vi "TH_Bladmögelvarning.vi"(4 "Bladmögelvarning":T1={"Tid (Timmar)"=5.0, "Grader (°C)"=15.0, "Fuktighet (%)"=80.0} {"Fuktighet (%)" min=0.0 max=100.0 format="%.1f"; "Grader (°C)" min=-25.0 max=85.0 format="%.1f"; "Tid (Timmar)" min=0.01 format="%.2f"}, 6 "Humidities In":dbl[](array[numeric]) format="%.2f", 7 "Temperatures In":dbl[](array[numeric]) format="%.2f") -> (3 "Bladmägelvarning (T/F)":bool)   [LabVIEW 2014]
panel:
  in  "Startflag":bool
  out "Starttid (sec)":dbl
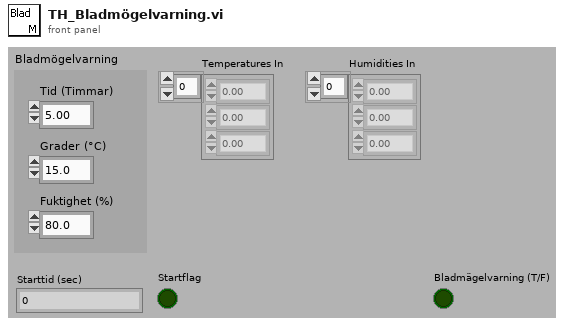
[diagram p1: front panel]
types:
  T1 = cluster{"Tid (Timmar)":dbl, "Grader (°C)":dbl, "Fuktighet (%)":dbl}
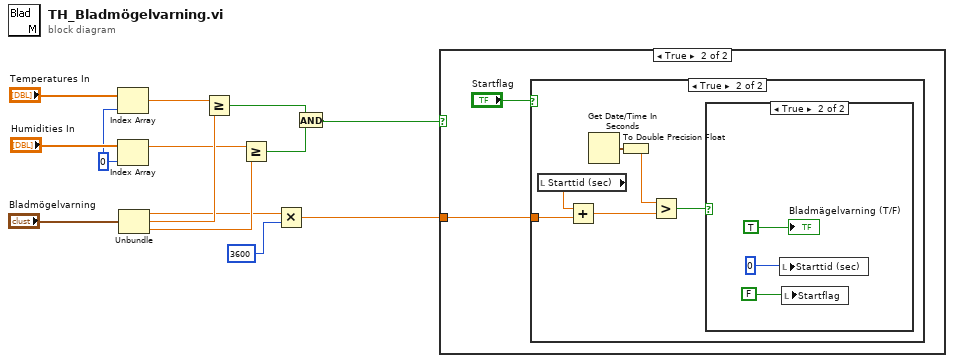
[diagram p0: block diagram]
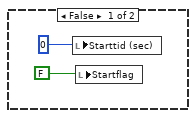
[diagram p2: hidden frame]
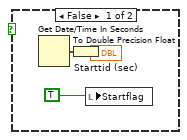
[diagram p3: hidden frame]
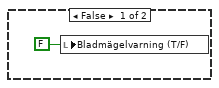
[diagram p4: hidden frame]
diagram:
  w12 = 0 ("Index")
  n1 = Index Array(array="Temperatures In", index=w12) -> (element=w10:dbl)
  n2 = Index Array(array="Humidities In", index=w12) -> (element=w8:dbl)
  n3 = Unbundle("Bladmögelvarning") -> ("Tid (Timmar)"=w3:dbl, "Grader (°C)"=w9:dbl, "Fuktighet (%)"=w7:dbl)
  n4 = Greater Or Equal?(x=w10, y=w9) -> (x >= y?=w6:bool)
  n5 = Greater Or Equal?(x=w8, y=w7) -> (x >= y?=w5:bool)
  n6 = Multiply(x=w3, y=3600) -> (x*y=w1:dbl)
  n7 = And(x=w6, y=w5) -> (x .and. y?=w4:bool)
  n8 = case shown="True" w4 {
    tunnel: w1 -> [_ w17]
    frame False {
      n9 = local write "Starttid (sec)"(0) -> ()
      n10 = local write "Startflag"(FALSE) -> ()
    }
    frame True {
      n11 = case shown="True" "Startflag" {
        tunnel: w17 -> [_ w27]
        frame False {
          n12 = Get Date/Time In Seconds() -> (seconds since 1Jan1904=w19:timestamp)
          n13 = To Double Precision Float(number=w19) -> (double precision float=→"Starttid (sec)":dbl)
          n14 = local write "Startflag"(TRUE) -> ()
        }
        frame True {
          n15 = local read "Starttid (sec)"() -> (w26:dbl)
          n16 = Add(x=w26, y=w27) -> (x+y=w25:dbl)
          n17 = Get Date/Time In Seconds() -> (seconds since 1Jan1904=w22:timestamp)
          n18 = To Double Precision Float(number=w22) -> (double precision float=w24:dbl)
          n19 = Greater?(x=w24, y=w25) -> (0:w23:bool)
          n20 = case shown="True" w23 {
            frame False {
              n21 = local write "Bladmägelvarning (T/F)"(FALSE) -> ()
            }
            frame True {
              n22 = local write "Starttid (sec)"(0) -> ()
              n23 = local write "Startflag"(FALSE) -> ()
              "Bladmägelvarning (T/F)" <- TRUE ("Bladmägelvarning (T/F)")
            }
          }
        }
      }
    }
  }
